vi "Screen Tools.vi"() -> ()   [LabVIEW 2020]
uses:
  <vilib>/Utility/miscctls.llb/LVBoundsTypeDef.ctl
panel:
  in  "工具栏:可见":bool=TRUE
  in  "前面板窗口:可调整大小":bool=TRUE
  in  "动作":T1(ring)
  in  "状态":T2(ring)
  in  "应用":bool
  out "边界":T3
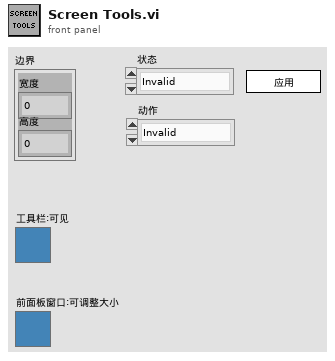
[diagram p1: front panel]
types:
  T1 = enum32{"Invalid", "Default", "Floating", "Floating/Auto-Hide", "Modal"}
  T2 = enum32{"Invalid", "Standard", "Closed", "Hidden", "Minimized", "Maximized"}
  T3 = typedef "LVBoundsTypeDef.ctl" = cluster{"Width":u32, "Height":u32}
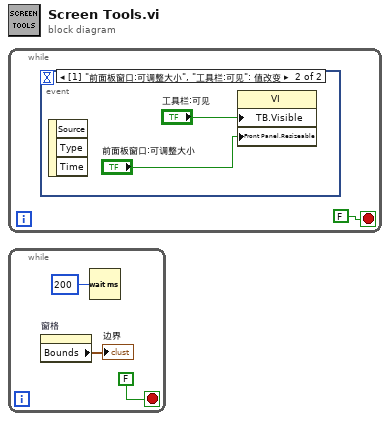
[diagram p0: block diagram]
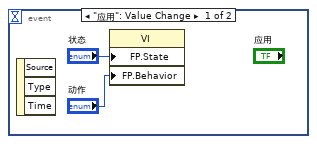
[diagram p2: hidden frame]
diagram:
  n1 = while {
    stop <- FALSE stop-if-true
    n2 = event shown="[1] \"前面板窗口:可调整大小\", \"工具栏:可见\": 值改变" {
      selector: _ -> [_ _]
      dyn-events: _ -> [_ _]
      timeout: _ -> [_ _]
      event "应用": Value Change {
        n3 = event-data() -> ()  [unwired: 1 in, 3 out]
        n4 = property class="VI"("FP.State"="状态", "FP.Behavior"="动作") -> ()  [unwired: 2 in, 2 out]
      }
      event "前面板窗口:可调整大小", "工具栏:可见": Value Change {
        n5 = event-data() -> ()  [unwired: 1 in, 3 out]
        n6 = property on="属性节点" class="VI"("TB.Visible"="工具栏:可见", "Front Panel.Resizeable"="前面板窗口:可调整大小") -> ()  [unwired: 2 in, 2 out]
      }
    }
  }
  n7 = while {
    stop <- FALSE stop-if-true
    n8 = property on="窗格" class="Pane"() -> ("Bounds"=→"边界":T3)  [unwired: 2 in, 2 out]
    n9 = Wait (ms)(milliseconds to wait=u32 200 ("等待时间（毫秒）")) -> ()  [unwired: 1 out]
  }
